vi "E700-Inverter Status Control.vi"(8 "error in (no error)":errorcluster, 10 "Direction Switch":bool, 11 "ON/OFF - Switch":bool) -> (0 "error out":errorcluster, 3 "Send Value":u16)   [LabVIEW 2020]
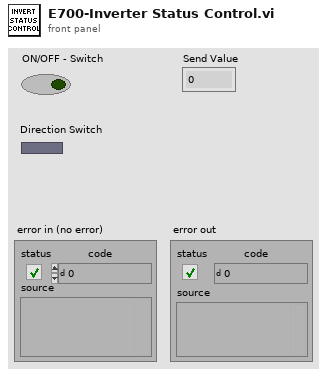
[diagram p1: front panel]
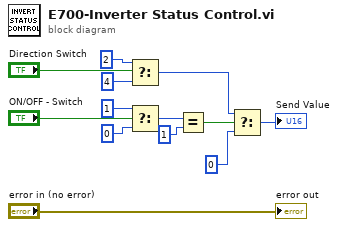
[diagram p0: block diagram]
diagram:
  n1 = Select(t=u16 2, s="Direction Switch", f=u16 4) -> (s? t:f=w9:u16)
  n2 = Select(t=u16 1, s="ON/OFF - Switch", f=u16 0) -> (s? t:f=w8:u16)
  n3 = Equal?(x=w8, y=u16 1) -> (x = y?=w11:bool)
  n4 = Select(t=w9, s=w11, f=u16 0) -> (s? t:f=→"Send Value":u16)
  "error out" <- "error in (no error)"
